vi "Do Core.vi"(8 "error in (no error)":errorcluster, 9 "Actor in":refnum<class "Actor.lvclass">, 11 "Reply Message":refnum<class "Get Connection List Msg.lvclass">) -> (0 "error out":errorcluster, 1 "Actor out":refnum<class "Actor.lvclass">, 2 "Reply":variant)   [LabVIEW 2017, in "Connection Listener.lvlib" / "Get Connection List Msg.lvclass"]
doc: "(<B>Filename</B>: Actor Framework.lvlib:Reply Msg.lvclass:Do Core.vi)\n\nDefines what an actor does when it receives <B>Reply Message</B>. This method also defines the <B>Reply</B> that is returned to the actor that sent <B>Reply Message</B>.\n\nBy default, this method does nothing, and <B>Reply</B> is the ancestor Message class. A child class must override this method to define behavior and specify a child of the Message class to return in the <B>Reply</B> output."
uses:
  Get Connection List Msg.lvclass
  <vilib>/ActorFramework/Actor/Actor.lvclass
  Connection Listener/Connection Listener.lvclass
  Applications/National Instruments/LabVIEW 2017 64-bit/vi.lib/ActorFramework/Actor/Actor.lvclass
  <vilib>/ActorFramework/Message Enqueuer/Message Enqueuer.lvclass
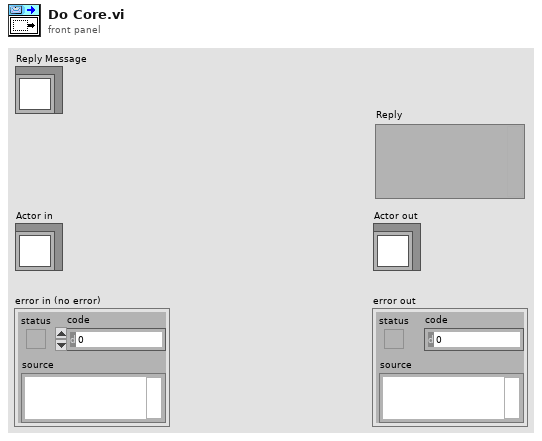
[diagram p1: front panel]
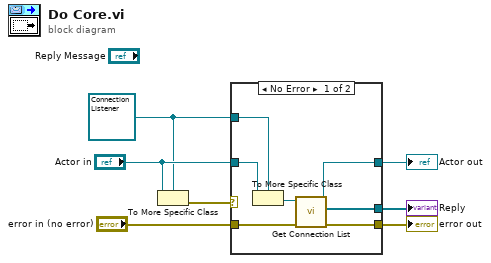
[diagram p0: block diagram]
diagram:
  w3 = refnum<class "Connection Listener.lvclass"> refnum ("Connection Listener.lvlib:Connection Listener.lvclass")
  n1 = To More Specific Class(target class=w3, reference="Actor in") -> (error out=w5:errorcluster)  [unwired: 1 in, 1 out]
  n2 = case shown="No Error" w5 {
    tunnel: "error in (no error)" -> [w11 w16]
    tunnel: [w10 w16] -> w6
    tunnel: "Actor in" -> [w14 w15]
    tunnel: w3 -> [w13 _]
    tunnel: [w9 w15] -> w2
    tunnel: [w8 _] -> w1
    frame No Error {
      n3 = To More Specific Class(target class=w13, reference=w14) -> (specific class reference=w12:refnum<class "Connection Listener.lvclass">)  [unwired: 1 in, 1 out]
      n4 = call "Get Connection List.vi"("error in (no error)"=w11, "Connection Listener in"=w12) -> ("error out"=w10:errorcluster, "ConnHandlers"=w8:refnum<class "Message Enqueuer.lvclass">[], "Connection Listener out"=w9:refnum<class "Connection Listener.lvclass">)  [unwired: 7 in]
    }
    frame Error {
    }
  }
  "error out" <- w6
  "Actor out" <- w2
  "Reply" <- w1
